vi "SetHintWithPriority.vi"(8 "No Error":errorcluster, 9 "Priority":T1, 10 "Value":string, 11 "Hint Name":T2) -> (0 "error out":errorcluster)   [LabVIEW 2024, in "SDL3.lvlib" / "Hints.lvlib"]
doc: "<B>Summary</B>\nSet a hint with a specific priority.\n\n<B>Remarks</B>\nThe priority controls the behavior when setting a hint that already has a value. Hints will replace existing hints of their priority and lower. Environment variables are considered to have override priority."
uses:
  HintName--combobox.ctl
  Hints.lvlib
  Lib/SDL3-32.dll
  Error/Error.lvlib
  HintPriority--enum.ctl
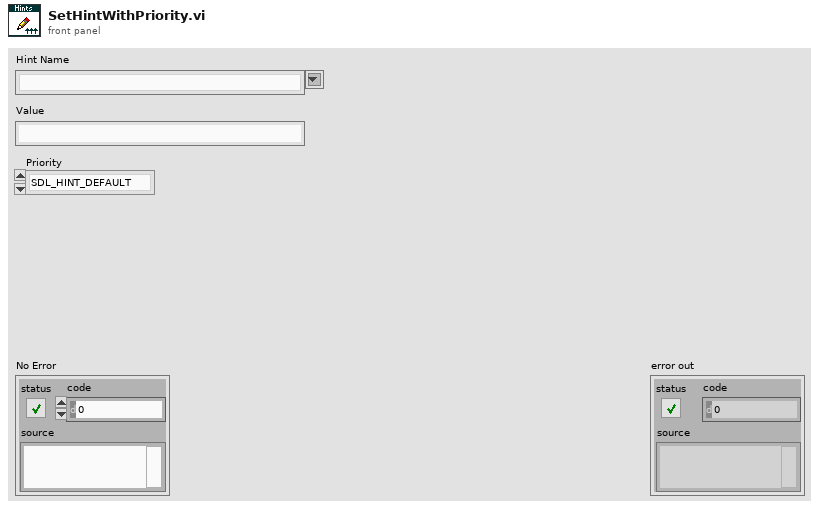
[diagram p1: front panel]
types:
  T1 = typedef "SDL3.lvlib/Hints.lvlib/HintPriority--enum.ctl" = enum32{"SDL_HINT_DEFAULT", "SDL_HINT_NORMAL", "SDL_HINT_OVERRIDE"}
  T2 = typedef "SDL3.lvlib/Hints.lvlib/HintName--combobox.ctl" = string
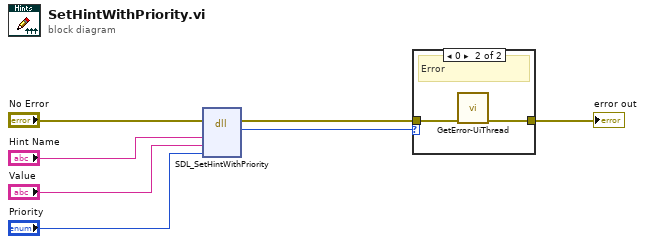
[diagram p0: block diagram]
diagram:
  n1 = dll-call lib="C:/Users/Thomas/Documents/Projects/LV-SDL3/Lib/SDL3-*.*" fn="SDL_SetHintWithPriority"(error in="No Error", "name"="Hint Name", "value"="Value", "hint_priority"="Priority") -> (error out=w3:errorcluster, "return type"=w2:i32)  [unwired: 5 in, 1 out]
  n2 = case shown="0" w2 {
    tunnel: w3 -> [w8 w10]
    tunnel: [w8 w9] -> w1
    frame Default {
      # "Ok"
    }
    frame 0 {
      # "Error"
      n3 = call "GetError-UiThread.vi"("No Error"=w10) -> ("error out"=w9:errorcluster)  [unwired: 10 in]
    }
  }
  "error out" <- w1
